vi "File.Open File or Folder.vi"(7 "IgnoreError":bool, 8 "Error In":errorcluster, 11 "Path":path) -> (0 "Error Out":errorcluster)   [LabVIEW 2024, in "EQMF.lvlib" / "File Utils.lvlib"]
doc: "This VI will open the file or folder specified by the input path.\n\nIf the file or folder does not exist, this VI will indicate an error."
uses:
  File Utils.lvlib
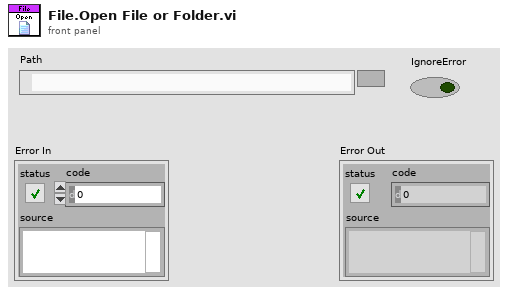
[diagram p1: front panel]
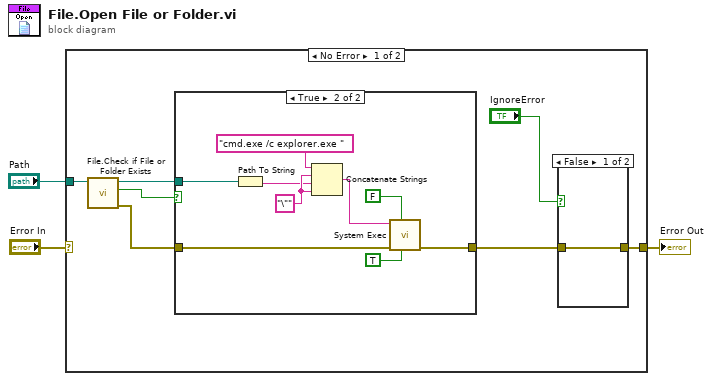
[diagram p0: block diagram]
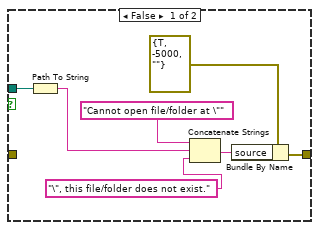
[diagram p3: hidden frame]
diagram:
  n1 = case shown="No Error" "Error In" {
    selector: "Error In" -> [_ w28]
    tunnel: [w4 w28] -> w3
    tunnel: "Path" -> [w10 _]
    frame No Error {
      n2 = call "File.Check if File or Folder Exists.vi"("Path"=w10) -> ("error out"=w7:errorcluster, "Exists"=w8:bool, "Dup Path"=w9:path)  [unwired: 6 in, 2 out]
      n3 = case shown="True" w8 {
        tunnel: w9 -> [w18 w25]
        tunnel: w7 -> [_ w20]
        tunnel: [w16 w19] -> w5
        frame False {
          n4 = Path To String(path=w18) -> (string=w12:string)
          n5 = Concatenate Strings("Cannot open file/folder at \"", w12, "\", this file/folder does not exist.") -> (w15:string)
          n6 = Bundle By Name(cluster=errorcluster {"status"=TRUE, "code"=-5000, "source"=""} ("error constant"), "source"=w15) -> (w16:errorcluster)
        }
        frame True {
          w22 = "\""
          n7 = Path To String(path=w25) -> (string=w21:string)
          n8 = Concatenate Strings("cmd.exe /c explorer.exe ", w22, w21, w22) -> (w24:string)
          n9 = call <vilib>:"System Exec.vi"("run minimized? (F)"=TRUE, "wait until completion? (T)"=FALSE, "error in (no error)"=w20, "command line"=w24) -> ("error out"=w19:errorcluster)  [unwired: 4 in, 3 out]
        }
      }
      n10 = case shown="False" "IgnoreError" {
        tunnel: w5 -> [w11 _]
        tunnel: [w11 _] -> w4
        frame False {
        }
        frame True {
        }
      }
    }
    frame Error {
    }
  }
  "Error Out" <- w3
